vi "DSF.Transceiver.UDP.Constants.Library Name.vi"() -> (3 "library name":string)   [LabVIEW 2017, in "DSF.Transceiver.UDP.lvlib" / "DSF.Transceiver.UDP.lvclass"]
uses:
  DSF.Transceiver.UDP.lvclass
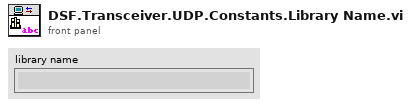
[diagram p1: front panel]
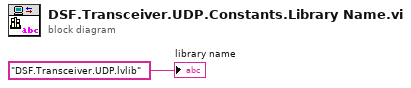
[diagram p0: block diagram]
diagram:
  "library name" <- "DSF.Transceiver.UDP.lvlib" ("base error code")
